vi "Condition Based on User Input (Triggering).vi"() -> ()   [LabVIEW 2020]
uses:
  <vilib>/DAQmx/read.llb/DAQmx Read (Analog 1D Wfm NChan NSamp).vi
  <vilib>/DAQmx/create/channels.llb/DAQmx Create Channel (AI-Voltage-Basic).vi
  <vilib>/DAQmx/configure/timing.llb/DAQmx Timing (Sample Clock).vi
  <vilib>/DAQmx/configure/trigger.llb/DAQmx Start Trigger (Digital Edge).vi
  <vilib>/DAQmx/miscellaneous.llb/DAQmx Fill In Error Info.vi
  <resource>/objmgr/daqmx.rc
panel:
  in  "Edge":u16(ring)=10280 items=["Rising"=10280, "Falling"=10171]
  in  "Digital Trigger Source":tag="/PCI-6221/PFI1"
  in  "Triggering Enabled?":bool
  out "Actual Sample Rate (Hz)":dbl
  in  "DAQmx Physical Channel":tag="PCI-6221/ai1"
  in  "Number of Samples":i32=100
  in  "Desired Sample Rate (Hz)":dbl=1000.0
  out "Waveform Graph":waveform(dbl)[](graph)
  # "Channel Settings"
  # "Acquired Data"
  # "______________________________________________"
  # "Timing Settings"
  # "______________________________________________"
  # "Trigger Settings"
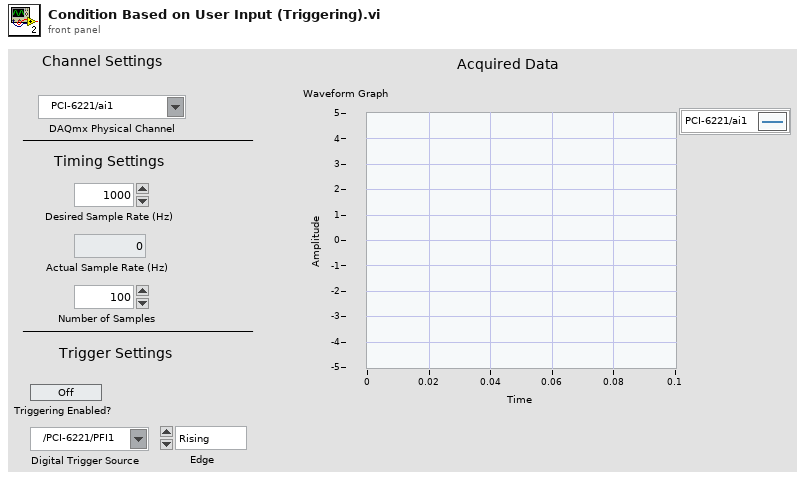
[diagram p1: front panel]
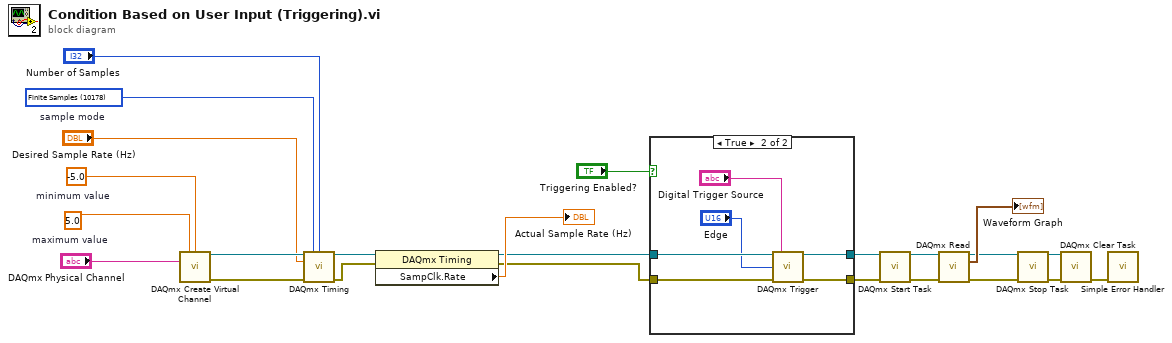
[diagram p0: block diagram]
diagram:
  w18 = 5.0  # maximum value
  w19 = -5.0  # minimum value
  w20 = 10178 items=["Finite Samples"=10178, "Continuous Samples"=10123, "Hardware Timed Single Point"=12522]  # sample mode
  n1 = call-poly <vilib>:"DAQmx Create Virtual Channel.vi"("maximum value"=w18, "minimum value"=w19, "physical channels"="DAQmx Physical Channel") -> ("task out"=w24:refnum<k21>, "error out"=w23:errorcluster)  [unwired: 11 in]
  n2 = call-poly <vilib>:"DAQmx Timing.vi"("task/channels in"=w24, "sample mode"=w20, "samples per channel"="Number of Samples", "rate"="Desired Sample Rate (Hz)", "error in"=w23) -> ("task out"=w21:refnum<k21>, "error out"=w22:errorcluster)  [unwired: 9 in]
  n3 = property class="DAQmx Timing"(reference=w21, error in=w22) -> (reference out=w12:refnum<k21>, error out=w11:errorcluster, "SampClk.Rate"=→"Actual Sample Rate (Hz)":dbl)
  n4 = case shown="True" "Triggering Enabled?" {
    tunnel: w12 -> [w26 w32]
    tunnel: w11 -> [w25 w31]
    tunnel: [w26 w29] -> w9
    tunnel: [w25 w28] -> w8
    frame False {
    }
    frame True {
      n5 = call-poly <vilib>:"DAQmx Trigger.vi"("task/channels in"=w32, "source"="Digital Trigger Source", "edge"="Edge", "error in"=w31) -> ("task out"=w29:refnum<k21>, "error out"=w28:errorcluster)  [unwired: 10 in]
    }
  }
  n6 = call <vilib>:"DAQmx Start Task.vi"("task/channels in"=w9, "error in"=w8) -> ("task out"=w7:refnum<k21>, "error out"=w6:errorcluster)  [unwired: 12 in]
  n7 = call-poly <vilib>:"DAQmx Read.vi"("task/channels in"=w7, "error in"=w6) -> ("task out"=w4:refnum<k21>, "data"=→"Waveform Graph":waveform(dbl)[], "error out"=w3:errorcluster)  [unwired: 11 in]
  n8 = call <vilib>:"DAQmx Stop Task.vi"("task/channels in"=w4, "error in"=w3) -> ("task out"=w2:refnum<k21>, "error out"=w1:errorcluster)  [unwired: 12 in]
  n9 = call <vilib>:"DAQmx Clear Task.vi"("task in"=w2, "error in"=w1) -> ("error out"=w17:errorcluster)  [unwired: 13 in]
  n10 = call <vilib>:"Simple Error Handler.vi"("error in (no error)"=w17) -> ()  [unwired: 4 in, 5 out]
